vi "StateLimeLight.vi"(0 "Master State In":T1(ring)) -> ()   [LabVIEW 2020]
doc: "This VI manages the LimeLight pipelines and LimeLight targeting LED mode."
uses:
  GlobalMiscellaneous.vi
  GlobalDriverStationData.vi
  GlobalPoseAndTargeting.vi
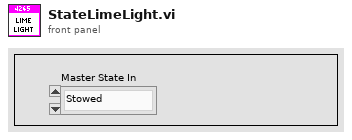
[diagram p1: front panel]
types:
  T1 = enum16{"Stowed", "Balancing", "Scoring", "Hoppering", "Ground", "Shelf"}
  T2 = enum16{"Boot Up", "Camera Override", "AprilTags", "Gamepiece Tracking"}
  T3 = enum16{"Side-by-Side", "PiP Main", "PiP Secondary"}
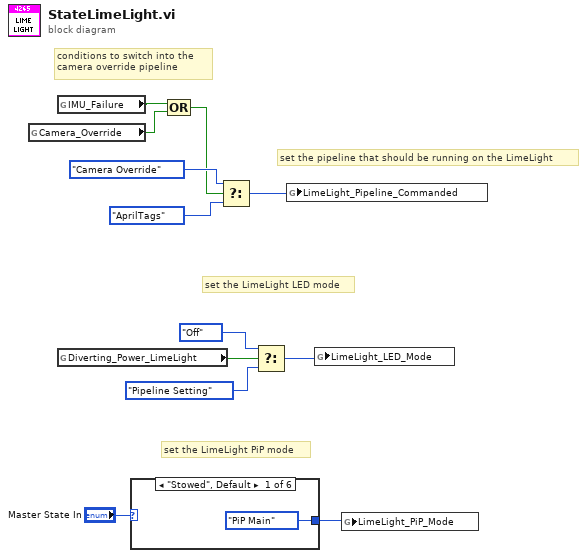
[diagram p0: block diagram]
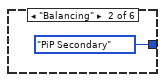
[diagram p2: hidden frame]
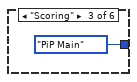
[diagram p3: hidden frame]
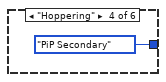
[diagram p4: hidden frame]
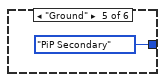
[diagram p5: hidden frame]
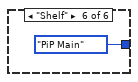
[diagram p6: hidden frame]
diagram:
  # "set the LimeLight PiP mode"
  # "set the LimeLight LED mode"
  # "conditions to switch into the \ncamera override pipeline"
  # "set the pipeline that should be running on the LimeLight"
  n1 = global read "GlobalDriverStationData.vi" "Camera_Override"() -> (w11:bool)
  n2 = global read "GlobalPoseAndTargeting.vi" "IMU_Failure"() -> (w12:bool)
  n3 = global read "GlobalMiscellaneous.vi" "Diverting_Power_LimeLight"() -> (w6:bool)
  n4 = case shown="\"Stowed\", Default" "Master State In" {
    tunnel: [T3."PiP Main" ("LimeLight_PiP_Mode") T3."PiP Secondary" ("LimeLight_PiP_Mode") T3."PiP Main" ("LimeLight_PiP_Mode") T3."PiP Secondary" ("LimeLight_PiP_Mode") T3."PiP Secondary" ("LimeLight_PiP_Mode") T3."PiP Main" ("LimeLight_PiP_Mode")] -> w1
    frame "Stowed", Default {
    }
    frame "Balancing" {
    }
    frame "Scoring" {
    }
    frame "Hoppering" {
    }
    frame "Ground" {
    }
    frame "Shelf" {
    }
  }
  n5 = Compound Arithmetic op=OR(w12, w11) -> (w9:bool)
  n6 = Select(t=T2."Camera Override", s=w9, f=T2."AprilTags") -> (s? t:f=w5:T2)
  n7 = Select(t=enum16{"Pipeline Setting", "Off", "Blink", "On"}."Off", s=w6, f=enum16{"Pipeline Setting", "Off", "Blink", "On"}."Pipeline Setting") -> (s? t:f=w4:enum16{"Pipeline Setting", "Off", "Blink", "On"})
  n8 = global write "GlobalMiscellaneous.vi" "LimeLight_Pipeline_Commanded"(w5) -> ()
  n9 = global write "GlobalMiscellaneous.vi" "LimeLight_LED_Mode"(w4) -> ()
  n10 = global write "GlobalMiscellaneous.vi" "LimeLight_PiP_Mode"(w1) -> ()
